vi "Get_Day_File_Summary.vi"(5 "End time":timestamp, 6 "Start time":timestamp, 8 "Data folder location":path) -> ()   [LabVIEW 2015]
uses:
  Anemometry/Anemometry Sub Vis/Globals/Constants_global.vi
  Anemometry/Anemometry Sub Vis/Globals/Preference_global.vi
panel:
  in  "Output Filename":path
  out "Names":string[](array[string])
  out "Summary":string[][](array[string])
  in  "Template":path
  out "Currenly reading":path
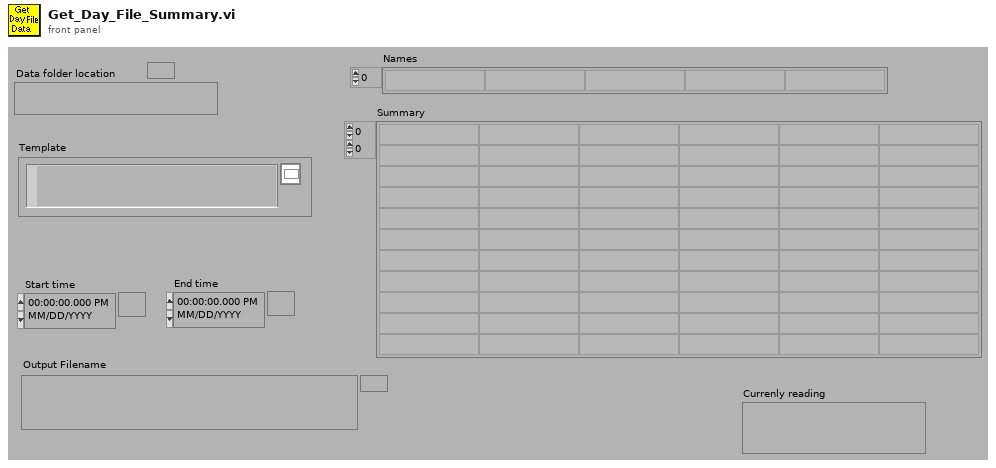
[diagram p1: front panel]
types:
  T1 = typedef "LVDateTimeRec.ctl" = cluster{"fractional second":dbl, "second":i32, "minute":i32, "hour":i32, "day of month":i32, "month":i32, "year":i32, "day of week":i32, "day of year":i32, "DST":i32}
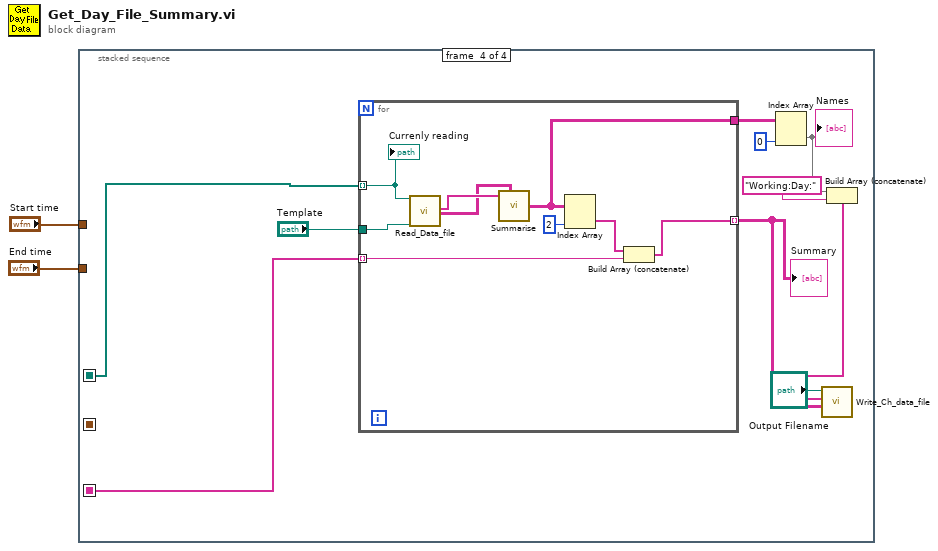
[diagram p0: block diagram]
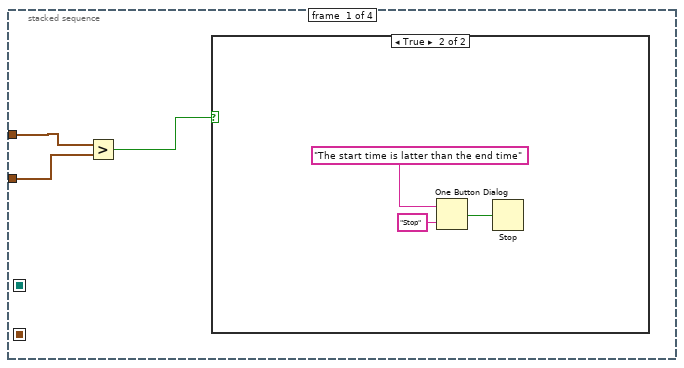
[diagram p2: hidden frame]
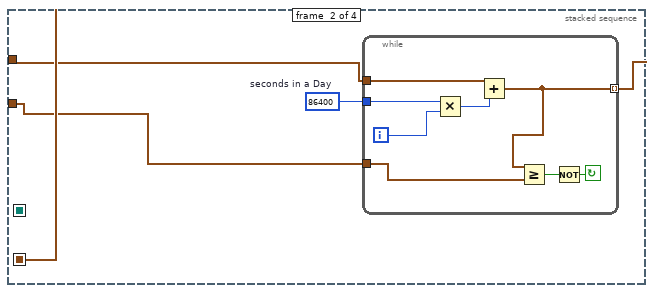
[diagram p4: hidden frame]
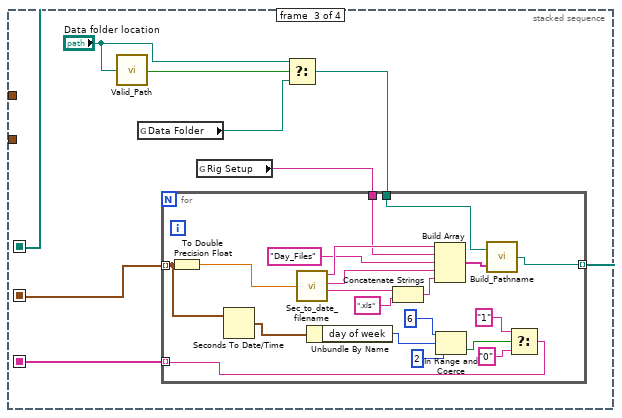
[diagram p5: hidden frame]
diagram:
  n1 = stacked-sequence {
    seq-local: [_ w12 _ _] -> [_ _ w28 _]
    seq-local: [_ _ w27 _] -> [_ _ _ w58]
    seq-local: [_ _ w21 _] -> [_ _ _ w54]
    tunnel: "End time" -> [w4 w9 _ _]
    tunnel: "Start time" -> [w3 w10 _ _]
    frame #0 {
      n2 = Greater?(x=w3, y=w4) -> (0:w5:bool)
      n3 = case shown="True" w5 {
        frame False {
        }
        frame True {
          n4 = One Button Dialog(message="The start time is latter than the end time", button name ("OK")="Stop") -> (true=w7:bool)
          n5 = Stop(stop? (T)=w7) -> ()
        }
      }
    }
    frame #1 {
      w11 = u32 86400  # seconds in a Day
      n6 = while {
        tunnel: [w13] -> w12 mode=indexing
        tunnel: w9 -> [w20]
        tunnel: w10 -> [w14]
        tunnel: w11 -> [w16]
        i -> [w17]
        stop <- w18 continue-if-true
        n7 = Multiply(x=w16, y=w17) -> (x*y=w15:u32)
        n8 = Add(x=w14, y=w15) -> (x+y=w13:timestamp)
        n9 = Greater Or Equal?(x=w13, y=w20) -> (x >= y?=w19:bool)
        n10 = Not(x=w19) -> (.not. x?=w18:bool)
      }
    }
    frame #2 {
      n11 = call "Valid_Path.vi"("Filename"="Data folder location") -> ("Valid Path?"=w26:bool)
      n12 = global read "Constants_global.vi" "Data Folder"() -> (w24:path)
      n13 = global read "Preference_global.vi" "Rig Setup"() -> (w22:string)
      n14 = Select(t="Data folder location", s=w26, f=w24) -> (s? t:f=w23:path)
      n15 = for {
        tunnel: w28 -> [w37] mode=indexing
        tunnel: w23 -> [w42]
        tunnel: [w39] -> w27 mode=indexing
        tunnel: w22 -> [w38]
        tunnel: [w30] -> w21 mode=indexing
        n16 = To Double Precision Float(number=w37) -> (double precision float=w40:dbl)
        n17 = Seconds To Date/Time(time stamp (now)=w37) -> (date time rec=w36:T1)  [unwired: 1 in]
        n18 = call "Sec_to_date_filename.vi"("seconds"=w40) -> ("Year"=w45:string, "Month"=w44:string, "Day"=w48:string)  [unwired: 1 out]
        n19 = Unbundle By Name(w36) -> ("day of week"=w35:i32)
        n20 = Concatenate Strings(w48, ".xls" ("string")) -> (w46:string)
        n21 = Build Array(w45, w38, "Day_Files" ("Input Element"), w44, w46) -> (w41:string[])
        n22 = In Range and Coerce(upper limit=6, x=w35, lower limit=2) -> (In Range?=w32:bool)  [unwired: 1 out]
        n23 = call "Build_Pathname.vi"("PathElements"=w41, "PathnameIn"=w42) -> ("AppendedPath"=w39:path)
        n24 = Select(t="1", s=w32, f="0" ("t")) -> (s? t:f=w30:string)
      }
    }
    frame #3 {
      n25 = for {
        tunnel: w58 -> [w67] mode=indexing
        tunnel: "Template" -> [w66]
        tunnel: [w59] -> w53 mode=indexing
        tunnel: [w62] -> w55
        tunnel: w54 -> [w60] mode=indexing
        n26 = call "Read_Data_file.vi"("Results file"=w67, "Template File"=w66) -> ("Ch names Out"=w65:string[], "Channel Values Out"=w64:string[][])  [unwired: 3 in, 13 out]
        n27 = call "Summarise.vi"("Channel Names"=w65, "Data"=w64) -> ("Summary"=w62:string[][])  [unwired: 3 in]
        n28 = Index Array(array=w62, index (col)=2 ("disabled index (col)")) -> (element=w61:string[])  [unwired: 1 in]
        n29 = Build Array (concatenate)(w61, w60) -> (w59:string[])
        "Currenly reading" <- w67
      }
      "Summary" <- w53
      n30 = Index Array(array=w55, index (col)=0 ("disabled index (col)")) -> (element=w52:string[])  [unwired: 1 in]
      "Names" <- w52
      n31 = Build Array (concatenate)(w52, "Working:Day:") -> (w50:string[])
      n32 = call "Write_Ch_data_file.vi"("Channel Values"=w53, "Channel names"=w50, "Filename"="Output Filename") -> ()  [unwired: 9 in]
    }
  }
